vi "Switch Action.vi"() -> ()   [LabVIEW 2016]
uses:
  <vilib>/rvi/Emulation/niFpgaGetClockAttributes.vi
  <vilib>/rvi/Emulation/niFpgaSctlEmulationGetInTimedLoop.vi
  <vilib>/rvi/Emulation/niFpgaEmulationReportErrorSimple.vi
  <vilib>/rvi/eio/common/nirviEmuTemplateMethod_errors.vi
  <vilib>/rvi/Emulation/niFpgaCriticalErrorInLSC.vi
  <vilib>/eio/EIONode/EIONode.xnode
panel:
  in  "stop":bool
  out "Virtual\n LED":bool
  in  "Virtual \nSwitch":bool
  out "DIO4":bool
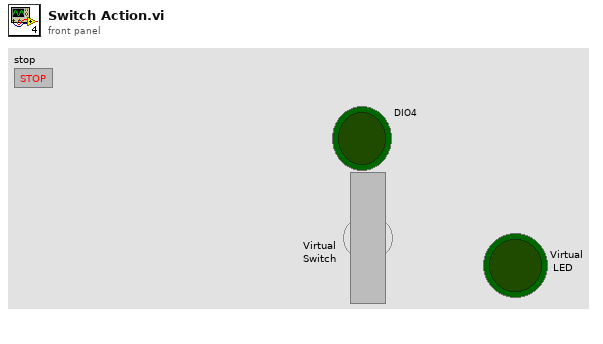
[diagram p1: front panel]
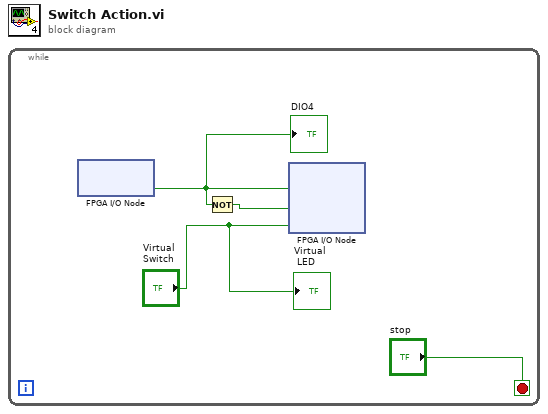
[diagram p0: block diagram]
diagram:
  n1 = while {
    stop <- "stop" stop-if-true
    n2 = xnode "FPGA I/O Node"() -> ("DIO12"=w3:bool)  [unwired: 1 in, 1 out]
    "DIO4" <- w3
    n3 = Not(x=w3) -> (.not. x?=w4:bool)
    n4 = xnode "FPGA I/O Node"("DIO4"=w3, "DIO5"=w4, "DIO6"="Virtual \nSwitch") -> ()  [unwired: 3 in, 3 out]
    "Virtual\n LED" <- "Virtual \nSwitch"
  }
